vi "_TangoAttributeEventHandler.vi"(3 "error in":errorcluster, 4 "timeout (ms)":i32=1000, 5 "attribute event ref.":T1) -> (0 "error out":errorcluster, 1 "attribute raw data":T2={"device name"="", "attribute name"="", "quality value"=0, "quality string"="", "timestamp"=0.0, "dim. x"=0, "dim. y"=0, "value"=[], "error code"=0, "error stack"=[], "data type"=36}, 2 "event timeout":bool)   [LabVIEW 2014, in "tango.lvlib"]
uses:
  tango.lvlib
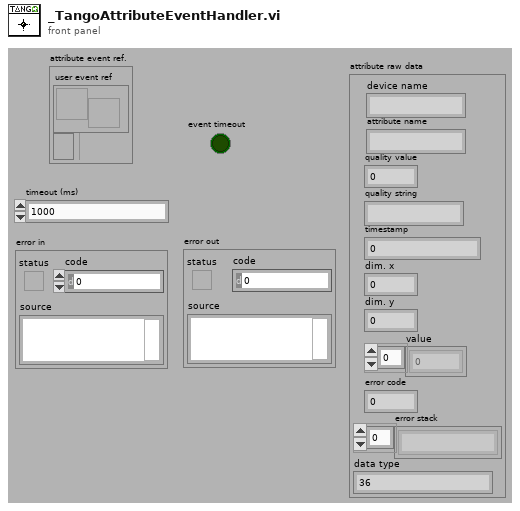
[diagram p1: front panel]
types:
  T1 = cluster{"user event ref":refnum<user-event>, "user event reg refnum":refnum<event-registration>}
  T2 = cluster{"device name":string, "attribute name":string, "quality value":i16, "quality string":string, "timestamp":dbl, "dim. x":i32, "dim. y":i32, "value":u8[], "error code":i32, "error stack":string[], "data type":u16}
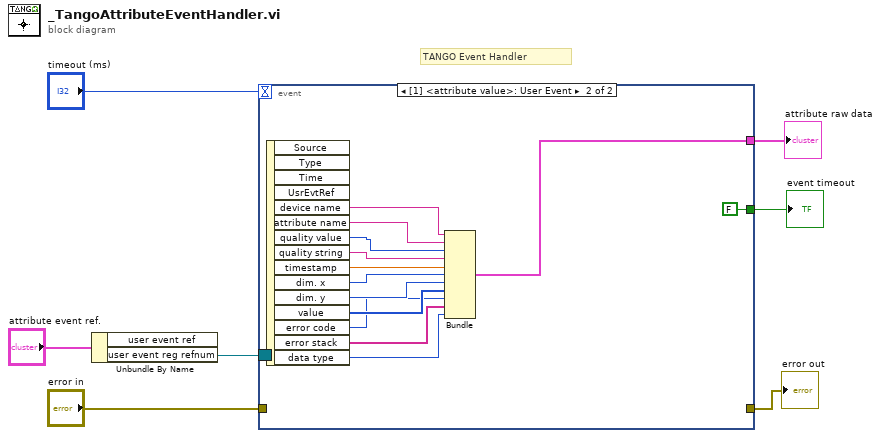
[diagram p0: block diagram]
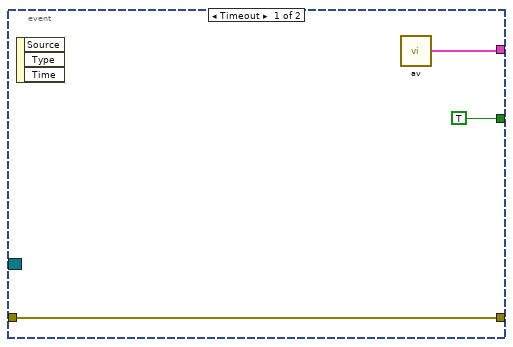
[diagram p2: hidden frame]
diagram:
  # "TANGO Event Handler"
  n1 = Unbundle By Name("attribute event ref.") -> ("user event reg refnum"=w2:refnum<event-registration>)  [unwired: 1 out]
  n2 = event shown="[1] <attribute value>: User Event" {
    selector: w2 -> [_ _]
    dyn-events: _ -> [_ _]
    timeout: "timeout (ms)" -> [_ _]
    tunnel: [TRUE FALSE] -> w7
    tunnel: [w8 w12] -> w4
    tunnel: "error in" -> [w9 _]
    tunnel: [w9 _] -> w5
    event Timeout {
      n3 = event-data() -> ()  [unwired: 1 in, 3 out]
      n4 = call "av.vi"() -> ("attribute value"=w8:T2)  [unwired: 6 in]
    }
    event User Event {
      n5 = event-data() -> ("device name"=w23:string, "attribute name"=w22:string, "quality value"=w21:i16, "quality string"=w20:string, "timestamp"=w19:dbl, "dim. x"=w18:i32, "dim. y"=w17:i32, "value"=w16:u8[], "error code"=w15:i32, "error stack"=w14:string[], "data type"=w13:u16)  [unwired: 1 in, 4 out]
      n6 = Bundle("device name"=w23, "attribute name"=w22, "quality value"=w21, "quality string"=w20, "timestamp"=w19, "dim. x"=w18, "dim. y"=w17, "value"=w16, "error code"=w15, "error stack"=w14, "data type"=w13) -> (w12:T2)  [unwired: 1 in]
    }
  }
  "event timeout" <- w7
  "error out" <- w5
  "attribute raw data" <- w4
